vi "Init Adapter.vi"(3 "Rack":u16, 5 "Slot":u16) -> (1 "ISO_CR":u8[](array[numeric]) format="%.0x")   [LabVIEW 2014, in "Simatic S7.lvlib"]
uses:
  Simatic S7.lvlib
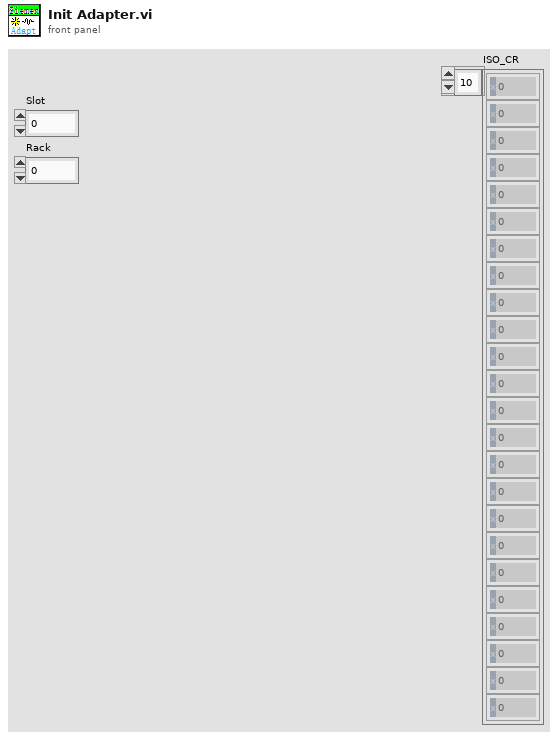
[diagram p1: front panel]
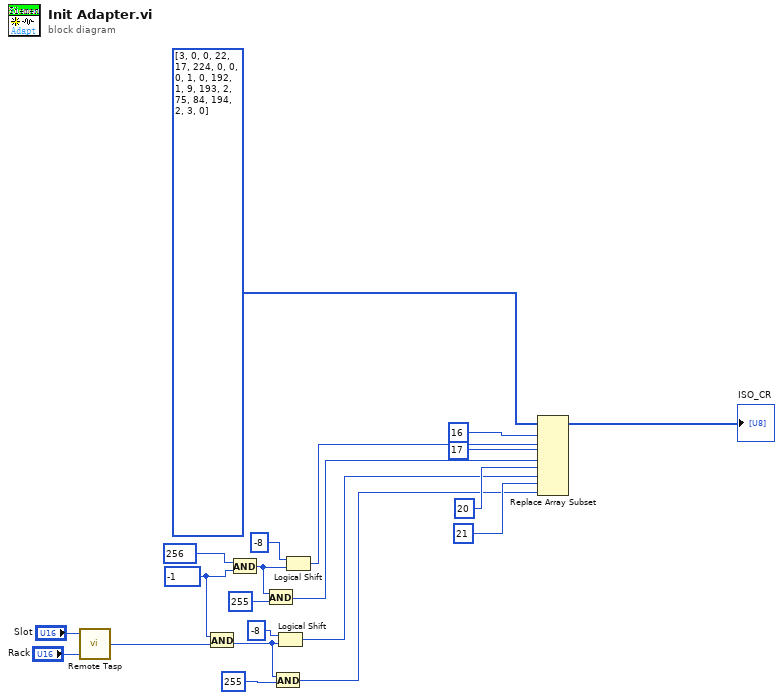
[diagram p0: block diagram]
diagram:
  w17 = i16 -1
  n1 = call "Remote Tasp.vi"("Rack"="Rack", "Slot"="Slot") -> ("RemoteTSAP"=w3:i16)  [unwired: 3 in]
  n2 = And(x=w17, y=w3) -> (x .and. y?=w15:i16)
  n3 = And(x=i16 256, y=w17) -> (x .and. y?=w19:i16)
  n4 = And(x=w19, y=255) -> (x .and. y?=w6:i32)
  n5 = And(x=w15, y=255) -> (x .and. y?=w4:i32)
  n6 = Logical Shift(y=i16 -8, x=w15) -> (x << y=w5:i16)
  n7 = Logical Shift(y=i16 -8, x=w19) -> (x << y=w7:i16)
  n8 = Replace Array Subset(array=u8[] [3, 0, 0, 22, 17, 224, 0, 0, 0, 1, 0, 192, 1, 9, 193, 2, 75, 84, 194, 2, 3, 0] ("添加的数组"), new element #1=w7, index #1=16 ("索引"), new element #2=w6, index #2=17 ("索引"), new element #3=w5, index #3=20 ("索引"), new element #4=w4, index #4=21 ("索引")) -> (→"ISO_CR":u8[])
